vi "LimitAI16_gen.vi"(0 "ClearLimit":bool, 1 "HighLimit":i16[](array[numeric])=[0, 0, 0, 0, 0, 0, 0, 0, 0, 0, 0, 0, 0, 0, 0, 0], 2 "UnscaledAI":i16[](array[numeric])=[0, 0, 0, 0, 0, 0, 0, 0, 0, 0, 0, 0, 0, 0, 0, 0], 5 "UnscaledLimitLowIn":u16, 7 "UnscaledLimitHighIn":u16, 9 "input valid":bool=TRUE, 11 "LowLimit":i16[](array[numeric])=[0, 0, 0, 0, 0, 0, 0, 0, 0, 0, 0, 0, 0, 0, 0, 0], 12 "LimitiEnabled":u16) -> (4 "UnscaledLimitLowOut":u16, 6 "UnscaledLimitHighOut":u16, 8 "LimitReached":bool, 10 "output valid":bool, 14 "feedback signals":cluster{"ready for input":bool})   [LabVIEW 2015]
doc: "This VI is created by the NI LabVIEW 2015 FPGA IP Builder.\n\nProject: ScaleAndLimit.lvproj\nTarget: FPGA Target (sbRIO-9607)/IP Builder\nBuild Specification: LimitAI16_src\nDirectives Item: LimitAI16_src\nTop-Level VI: C:\\LabVIEWPowerElectronicsControl\\ScaleAndLimit\\dev\\Core\\IPBuilder\\LimitAI16_src.vi\n\nQuick Device Utilization Estimate\n--------------------------------------------\nSlice Registers: 0.9% (957 out of 106400)\nSlice LUTs: 2.6% (1399 out of 53200)\nDSP48s: 0.0% (0 out of 220)\nBlock RAMs: 0.0% (0 out of 280)\n\nQuick Performance Estimate\n--------------------------------------------\nClock rate (MHz): 137.74\nInitiation interval (cycles): 18\nPipeline type: Not pipelined\nMinimum latency: 17\nMaximum latency: 17"
uses:
  <vilib>/rvi/IPIntegrationNode/IPINode_Typedef/niFpgaIPINodeSupportedFamilies.ctl
  <vilib>/rvi/IPIntegrationNode/IPINode_Utilities/niFpgaIPINodeSimCore.vi
  <vilib>/rvi/IPIntegrationNode/IPINode_Xnode/niFpgaIPINode.xnode
  LimitAI16_gen Support/IPBlockSimFiles/xsim.dir/mDE216D88_topH/xsimk87039E4BEC3D41B4A9B293BCBAB5F068.dll
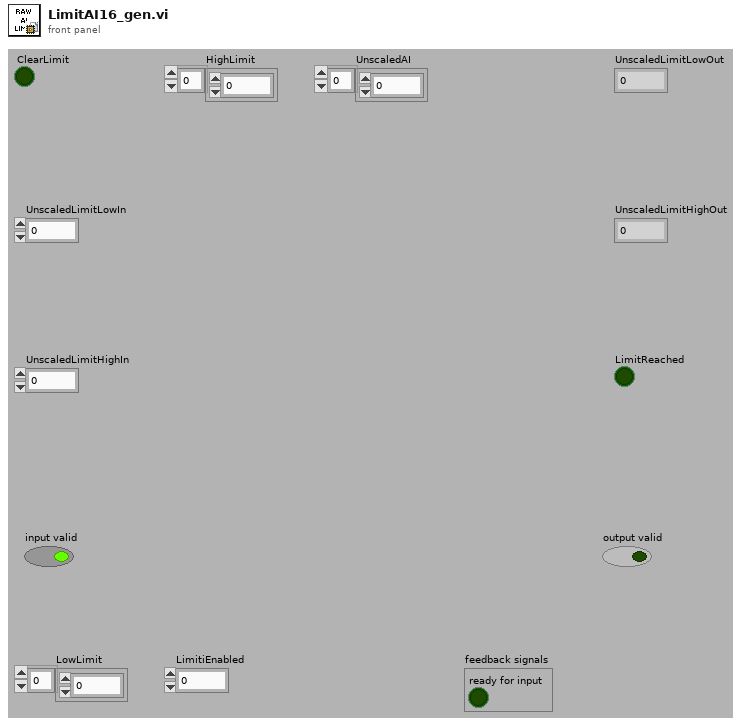
[diagram p1: front panel]
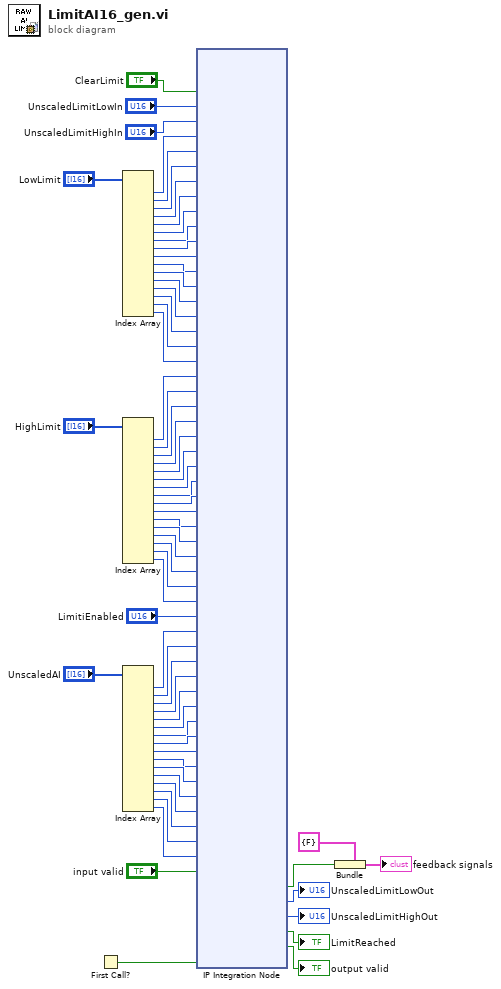
[diagram p0: block diagram]
diagram:
  n1 = First Call?() -> (First Call?: T/F=w64:bool)
  n2 = Index Array(array="LowLimit") -> (element #1=w37:i16, element #2=w38:i16, element #3=w39:i16, element #4=w40:i16, element #5=w41:i16, element #6=w42:i16, element #7=w43:i16, element #8=w44:i16, element #9=w45:i16, element #10=w46:i16, element #11=w47:i16, element #12=w48:i16, element #13=w49:i16, element #14=w50:i16, element #15=w51:i16, element #16=w52:i16)  [unwired: 16 in]
  n3 = Index Array(array="HighLimit") -> (element #1=w21:i16, element #2=w22:i16, element #3=w23:i16, element #4=w24:i16, element #5=w25:i16, element #6=w26:i16, element #7=w27:i16, element #8=w28:i16, element #9=w29:i16, element #10=w30:i16, element #11=w31:i16, element #12=w32:i16, element #13=w33:i16, element #14=w34:i16, element #15=w35:i16, element #16=w36:i16)  [unwired: 16 in]
  n4 = Index Array(array="UnscaledAI") -> (element #1=w4:i16, element #2=w5:i16, element #3=w6:i16, element #4=w7:i16, element #5=w8:i16, element #6=w9:i16, element #7=w10:i16, element #8=w11:i16, element #9=w12:i16, element #10=w13:i16, element #11=w14:i16, element #12=w15:i16, element #13=w16:i16, element #14=w17:i16, element #15=w18:i16, element #16=w19:i16)  [unwired: 16 in]
  n5 = xnode "IP Integration Node"("p_12_ClearLimit"="ClearLimit", "p_11_UnscaledLimitLowIn"="UnscaledLimitLowIn", "p_9_UnscaledLimitHighIn"="UnscaledLimitHighIn", "p_7_LowLimit_0"=w37, "p_7_LowLimit_1"=w38, "p_7_LowLimit_2"=w39, "p_7_LowLimit_3"=w40, "p_7_LowLimit_4"=w41, "p_7_LowLimit_5"=w42, "p_7_LowLimit_6"=w43, "p_7_LowLimit_7"=w44, "p_7_LowLimit_8"=w45, "p_7_LowLimit_9"=w46, "p_7_LowLimit_10"=w47, "p_7_LowLimit_11"=w48, "p_7_LowLimit_12"=w49, "p_7_LowLimit_13"=w50, "p_7_LowLimit_14"=w51, "p_7_LowLimit_15"=w52, "p_5_HighLimit_0"=w21, "p_5_HighLimit_1"=w22, "p_5_HighLimit_2"=w23, "p_5_HighLimit_3"=w24, "p_5_HighLimit_4"=w25, "p_5_HighLimit_5"=w26, "p_5_HighLimit_6"=w27, "p_5_HighLimit_7"=w28, "p_5_HighLimit_8"=w29, "p_5_HighLimit_9"=w30, "p_5_HighLimit_10"=w31, "p_5_HighLimit_11"=w32, "p_5_HighLimit_12"=w33, "p_5_HighLimit_13"=w34, "p_5_HighLimit_14"=w35, "p_5_HighLimit_15"=w36, "p_1_LimitiEnabled"="LimitiEnabled", "p_0_UnscaledAI_0"=w4, "p_0_UnscaledAI_1"=w5, "p_0_UnscaledAI_2"=w6, "p_0_UnscaledAI_3"=w7, "p_0_UnscaledAI_4"=w8, "p_0_UnscaledAI_5"=w9, "p_0_UnscaledAI_6"=w10, "p_0_UnscaledAI_7"=w11, "p_0_UnscaledAI_8"=w12, "p_0_UnscaledAI_9"=w13, "p_0_UnscaledAI_10"=w14, "p_0_UnscaledAI_11"=w15, "p_0_UnscaledAI_12"=w16, "p_0_UnscaledAI_13"=w17, "p_0_UnscaledAI_14"=w18, "p_0_UnscaledAI_15"=w19, "input_valid"="input valid", "first_call"=w64) -> ("ready_for_input"=w61:bool, "p_15_UnscaledLimitLowOut"=→"UnscaledLimitLowOut":u16, "p_10_UnscaledLimitHighOut"=→"UnscaledLimitHighOut":u16, "p_8_LimitReached"=→"LimitReached":bool, "output_valid"=→"output valid":bool)  [unwired: 2 in]
  n6 = Bundle ("Bundle_feedback")(cluster=cluster{"ready for input":bool} {"ready for input"=FALSE}, "ready for input"=w61) -> (→"feedback signals":cluster{"ready for input":bool})
